vi "take image.vi"(6 "Voltage":dbl, 7 "Exposure time":dbl, 9 "Busy out":refnum<k21>, 10 "Exp In":refnum<k21>, 11 "Galvo":refnum<k21>) -> ()   [LabVIEW 2019]
uses:
  <vilib>/DAQmx/write.llb/DAQmx Write (Digital Bool 1Line 1Point).vi
  <vilib>/DAQmx/write.llb/DAQmx Write (Analog DBL 1Chan 1Samp).vi
  <vilib>/DAQmx/read.llb/DAQmx Read (Digital Bool 1Line 1Point).vi
  <vilib>/DAQmx/miscellaneous.llb/DAQmx Fill In Error Info.vi
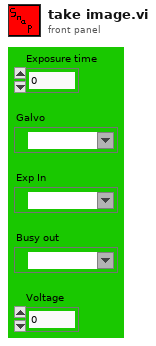
[diagram p1: front panel]
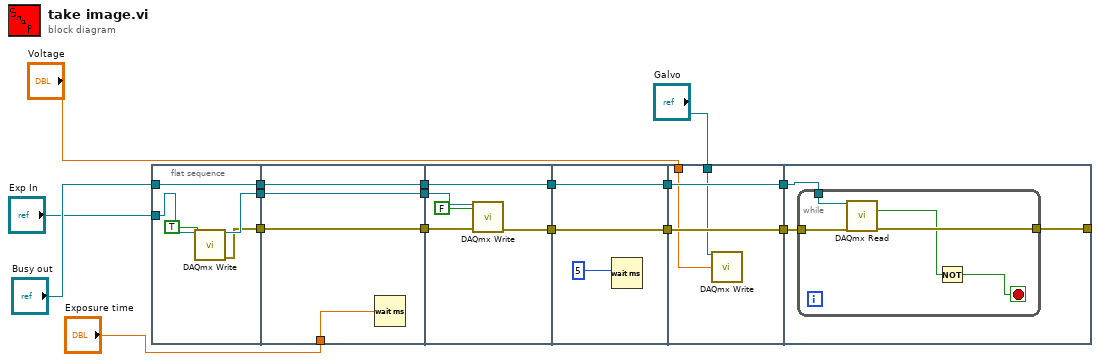
[diagram p0: block diagram]
diagram:
  n1 = flat-sequence {
    tunnel: [w21] -> w17
    tunnel: [w20] -> w16
    tunnel: "Busy out" -> [w19]
    tunnel: [w19] -> w15
    tunnel: "Exp In" -> [w18]
    tunnel: w17 -> [w26]
    tunnel: [w26] -> w14
    tunnel: w16 -> [w24]
    tunnel: [w25] -> w13
    tunnel: w15 -> [w25]
    tunnel: [w24] -> w12
    tunnel: "Exposure time" -> [w23]
    tunnel: w14 -> [w31]
    tunnel: [w29] -> w4
    tunnel: w13 -> [w29]
    tunnel: w12 -> [w28]
    tunnel: [w27] -> w2
    tunnel: w4 -> [w34]
    tunnel: [w34] -> w3
    tunnel: w2 -> [w33]
    tunnel: [w33] -> w1
    tunnel: w3 -> [w38]
    tunnel: [w38] -> w11
    tunnel: w1 -> [w37]
    tunnel: [w37] -> w10
    tunnel: "Voltage" -> [w36]
    tunnel: "Galvo" -> [w35]
    tunnel: w11 -> [w41]
    tunnel: w10 -> [w40]
    tunnel: [w39] -> _
    frame #0 {
      n2 = call-poly <vilib>:"DAQmx Write.vi"("task/channels in"=w18, "data"=TRUE) -> ("task out"=w21:refnum<k21>, "error out"=w20:errorcluster)  [unwired: 11 in, 1 out]
    }
    frame #1 {
      n3 = Wait (ms)(milliseconds to wait=w23) -> ()  [unwired: 1 out]
    }
    frame #2 {
      n4 = call-poly <vilib>:"DAQmx Write.vi"("task/channels in"=w31, "data"=FALSE, "error in"=w28) -> ("error out"=w27:errorcluster)  [unwired: 10 in, 2 out]
    }
    frame #3 {
      n5 = Wait (ms)(milliseconds to wait=5) -> ()  [unwired: 1 out]
    }
    frame #4 {
      n6 = call-poly <vilib>:"DAQmx Write.vi"("task/channels in"=w35, "data"=w36) -> ()  [unwired: 11 in, 3 out]
    }
    frame #5 {
      n7 = while {
        tunnel: w41 -> [w46]
        tunnel: w40 -> [w45]
        tunnel: [w44] -> w39
        stop <- w43 stop-if-true
        n8 = call-poly <vilib>:"DAQmx Read.vi"("task/channels in"=w46, "error in"=w45) -> ("data"=w42:bool, "error out"=w44:errorcluster)  [unwired: 11 in, 1 out]
        n9 = Not(x=w42) -> (.not. x?=w43:bool)
      }
    }
  }
